vi "ElevatorSim_GetPositionMeters.vi"(11 "ElevatorSim":T1={"LinearSystemSim"={"m_Plant"={"m_A"=[], "m_B"=[], "m_C"=[], "m_D"=[], "States"=0, "Inputs"=0, "Outputs"=0}, "m_X"=[], "m_Y"=[], "m_U"=[], "MeasureStdDev"=[]}, "GearBox"={"nominalVoltage_Volts"=0.0, "StallTorque_NM"=0.0, "StallCurrent_Amps"=0.0, "FreeCurrent_Amps"=0.0, "FreeSpeed_RadPerSec"=0.0, "R_Ohms"=0.0, "KvINV_RadPerSecPerVolt"=0.0, "Kt_NMPerAmp"=0.0, "L_H"=0.0, "Jr_KgM2"=0.0}, "Gearing"=0.0, "DrumRadius_M"=0.0, "MinHeight_M"=0.0, "MaxHeight_M"=0.0, "CarriageMass_Kg"=0.0, "SimulateGravity"=TRUE} {"GearBox"."Jr_KgM2" format="%13.5p"; "GearBox"."L_H" format="%13.5p"; "GearBox"."Kt_NMPerAmp" format="%13.5p"; "GearBox"."KvINV_RadPerSecPerVolt" format="%13.5p"; "GearBox"."R_Ohms" format="%13.5p"; "GearBox"."FreeSpeed_RadPerSec" format="%13.5p"; "GearBox"."FreeCurrent_Amps" format="%13.5p"; "GearBox"."StallCurrent_Amps" format="%13.5p"; "GearBox"."StallTorque_NM" format="%13.5p"; "GearBox"."nominalVoltage_Volts" format="%13.5p"}) -> (3 "Position_Meters":dbl)   [LabVIEW 2019, in "Trajectory_Library.lvlib"]
doc: "Returns the position of the elevator.\n \nInputs:\n - ElevatorSim -- Data cluster\n\nOutputs:\n - Position_Meters -- The position of the elevator. (Meters)"
uses:
  Trajectory_Library.lvlib
  TypeDef/LINEAR_SYSTEM.ctl
  <vilib>/Analysis/Matrix/Datatypes/RealMatrix.ctl
  <vilib>/Analysis/Matrix/NI_Matrix.lvlib
  TypeDef/DCMOTOR.CTL
  TypeDef/LINEAR_SYSTEM_SIM.ctl
  TypeDef/ELEVATOR_SIM.ctl
panel:
  # "<States, 1>"
  # "<Outputs, 1>"
  # "<Inputs, 1>"
  # "<Outputs, 1>"
  # "<States,States>"
  # "<States,Inputs>"
  # "<Outputs,States>"
  # "<Outputs,Inputs>"
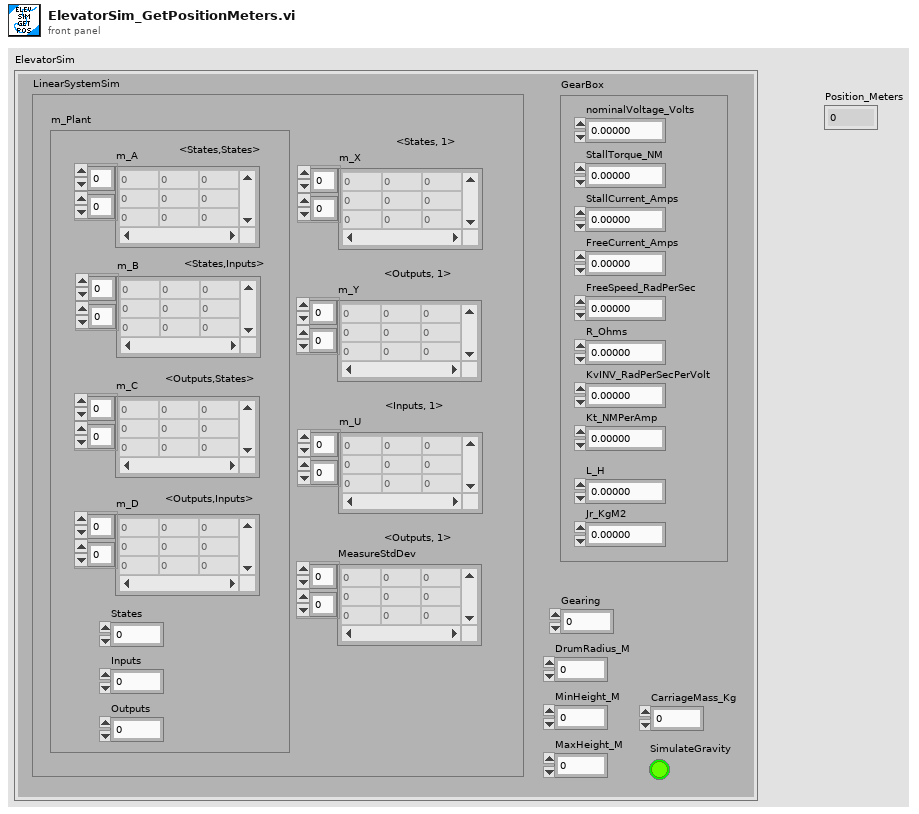
[diagram p1: front panel]
types:
  T1 = typedef "Trajectory_Library.lvlib/ELEVATOR_SIM.ctl" = cluster{"LinearSystemSim":T2, "GearBox":T5, "Gearing":dbl, "DrumRadius_M":dbl, "MinHeight_M":dbl, "MaxHeight_M":dbl, "CarriageMass_Kg":dbl, "SimulateGravity":bool}
  T2 = typedef "Trajectory_Library.lvlib/LINEAR_SYSTEM_SIM.ctl" = cluster{"m_Plant":T3, "m_X":T4, "m_Y":T4, "m_U":T4, "MeasureStdDev":T4}
  T3 = typedef "Trajectory_Library.lvlib/LINEAR_SYSTEM.ctl" = cluster{"m_A":T4, "m_B":T4, "m_C":T4, "m_D":T4, "States":i32, "Inputs":i32, "Outputs":i32}
  T4 = typedef "NI_Matrix.lvlib/RealMatrix.ctl" = dbl[][]
  T5 = typedef "Trajectory_Library.lvlib/DCMOTOR.CTL" = cluster{"nominalVoltage_Volts":dbl, "StallTorque_NM":dbl, "StallCurrent_Amps":dbl, "FreeCurrent_Amps":dbl, "FreeSpeed_RadPerSec":dbl, "R_Ohms":dbl, "KvINV_RadPerSecPerVolt":dbl, "Kt_NMPerAmp":dbl, "L_H":dbl, "Jr_KgM2":dbl}
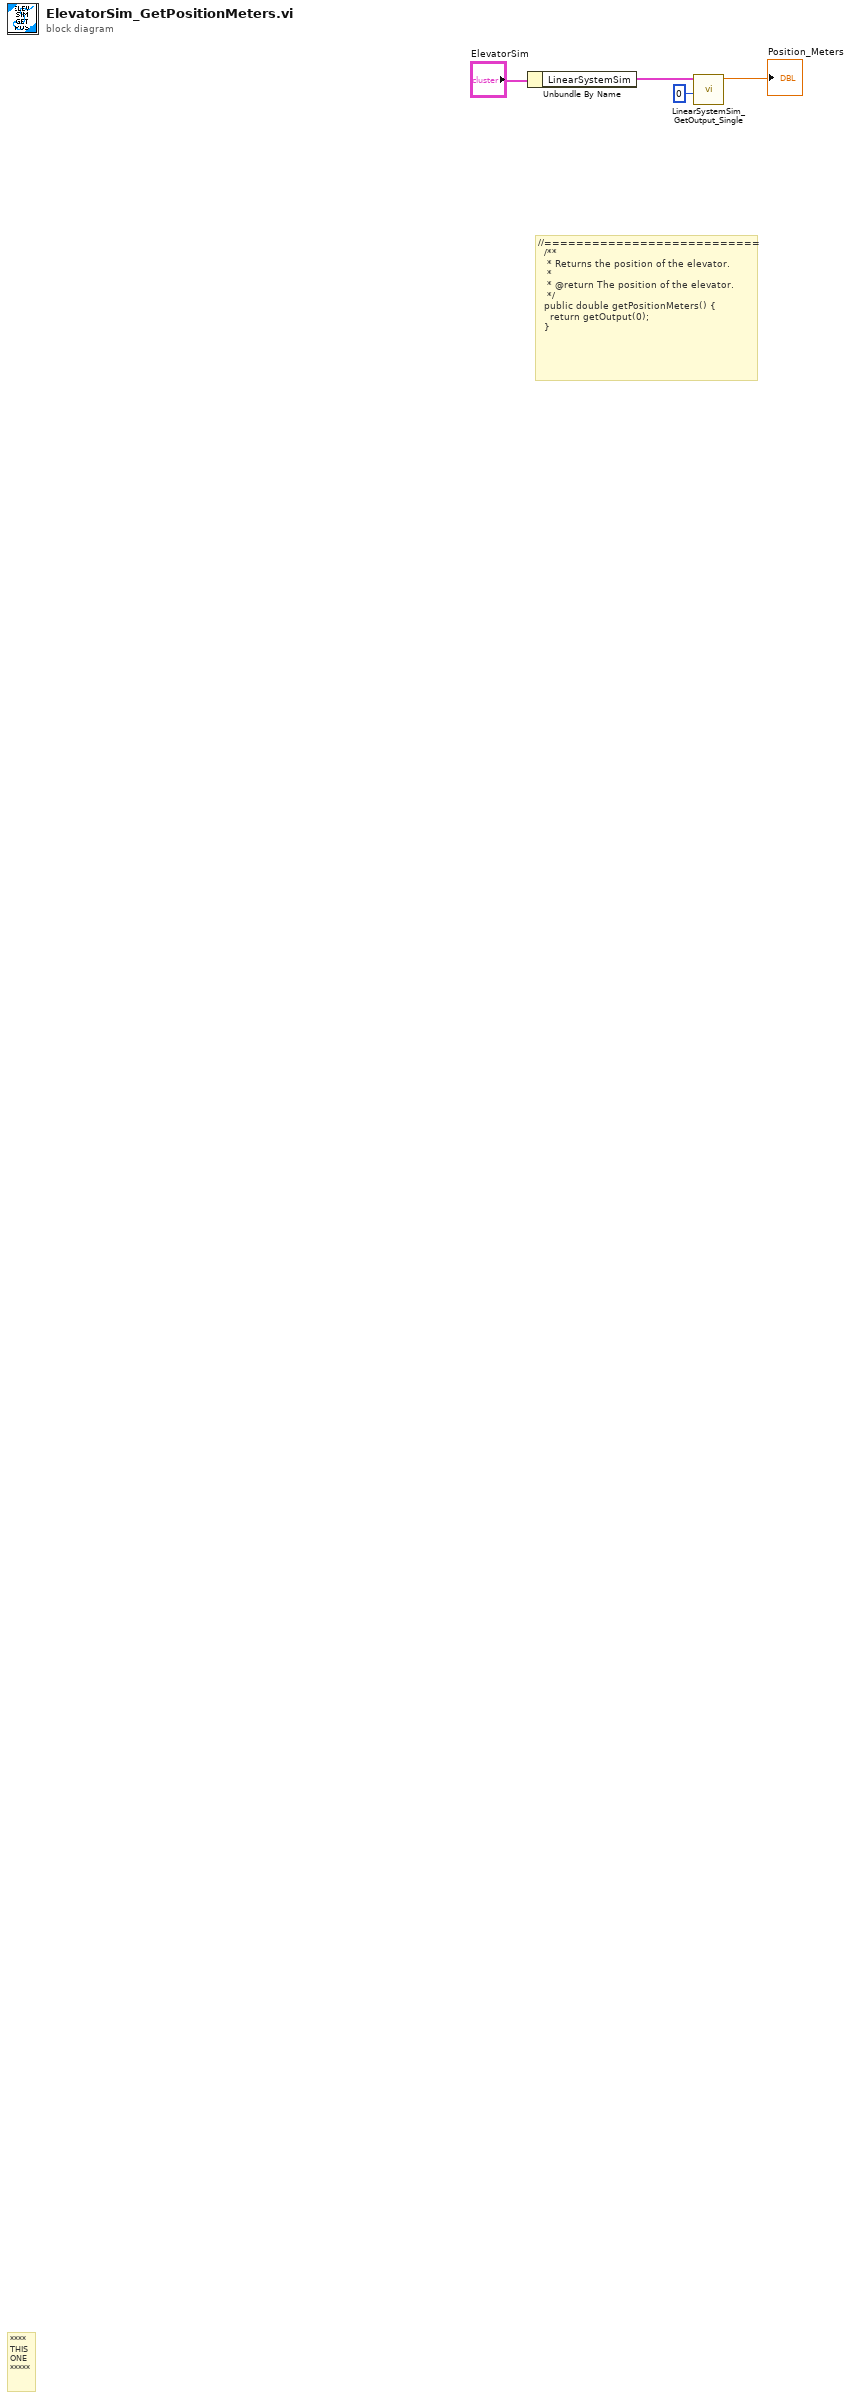
[diagram p0: block diagram]
diagram:
  # "//===========================\n  /**\n   * Returns the position of the elevator.\n   *\n   * @return The position of the elevator.\n   */\n  public double getPositionMeters() {\n    return getOutput(0);\n  }"
  # "****\nTHIS\nONE\n*****"
  n1 = Unbundle By Name("ElevatorSim") -> ("LinearSystemSim"=w3:T2)
  n2 = call "LinearSystemSim_GetOutput_Single.vi"("Row"=0, "LinearSysemSim"=w3) -> ("Output"=→"Position_Meters":dbl)  [unwired: 9 in]
